vi "FindMessageSet.vi"(7 "Actor":refnum<class "Actor.lvclass">) -> (3 "MessageSet":T1)   [LabVIEW 2020, in "_Template.lvlib" / "{{Actor}}.lvlib" / "Actor.lvclass"]
uses:
  Actor.lvclass
  jettl/jettl/Message/Message.lvclass
  Actor.lvclass/Actor.ctl
  jettl/jettl/jettl.lvlib
  jettl/jettl/MessageSet.ctl
panel:
  # "This front panel should not be manipulated."
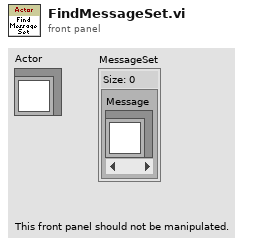
[diagram p1: front panel]
types:
  T1 = typedef "jettl.lvlib/MessageSet.ctl" = set{refnum<class "Message.lvclass">}
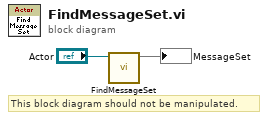
[diagram p0: block diagram]
diagram:
  # "This block diagram should not be manipulated."
  n1 = call "FindMessageSet.vi"("ConcreteActor.lvclass"="Actor") -> ("MessageSet"=→"MessageSet":T1)  [unwired: 10 in]
